vi "Read Waveform Array.vi"(8 "error in (no error)":errorcluster, 11 "Waveform Array Result in":refnum<class "Waveform Array Result.lvclass">) -> (0 "error out":errorcluster, 2 "Waveform Array":waveform(dbl)[](array[waveform]), 3 "Waveform Array Result out":refnum<class "Waveform Array Result.lvclass">)   [LabVIEW 2015, in "Waveform Array Result.lvclass"]
uses:
  Waveform Array Result.lvclass
  Waveform Array Result.lvclass/Waveform Array Result.ctl
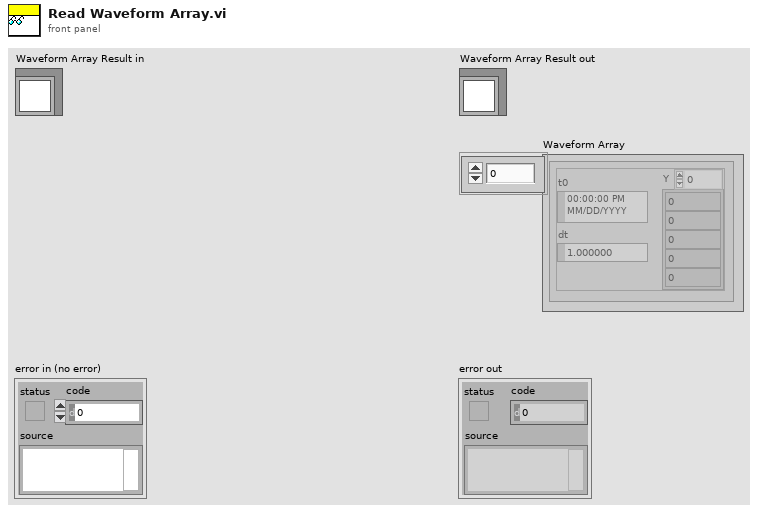
[diagram p1: front panel]
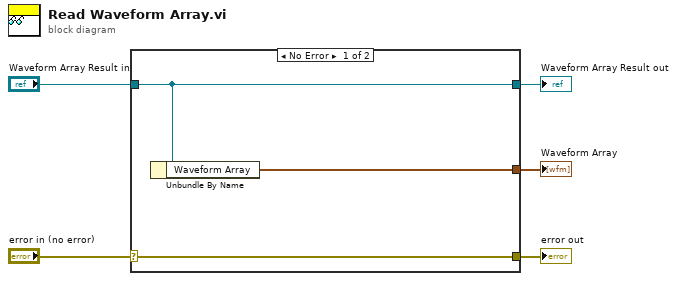
[diagram p0: block diagram]
diagram:
  n1 = case shown="No Error" "error in (no error)" {
    selector: "error in (no error)" -> [w8 w9]
    tunnel: [w8 w9] -> w4
    tunnel: [w7 w10] -> w2
    tunnel: "Waveform Array Result in" -> [w7 w10]
    tunnel: [w6 _] -> w1
    frame No Error {
      n2 = Unbundle By Name(w7) -> ("Waveform Array"=w6:waveform(dbl)[])
    }
    frame Error {
    }
  }
  "error out" <- w4
  "Waveform Array Result out" <- w2
  "Waveform Array" <- w1
